vi "Wait Single With Memory.vi"(8 "error in (no error)":errorcluster, 9 "Timeout in ms (-1)":i32=-1, 10 "Ignore previous (F)":bool, 11 "Notifier in":refnum<class "Notifier.lvclass">) -> (0 "error out":errorcluster, 1 "Timed out?":bool, 2 "Data Notification":refnum<class "Data.lvclass">, 3 "Notifier out":refnum<class "Notifier.lvclass">)   [LabVIEW 2020, in "Data.lvlib" / "Notifier.lvclass"]
doc: "Wait on notification from a single notifier with notifier history."
uses:
  Notifier.lvclass
  Data.lvclass
  Notifier.lvclass/Notifier.ctl
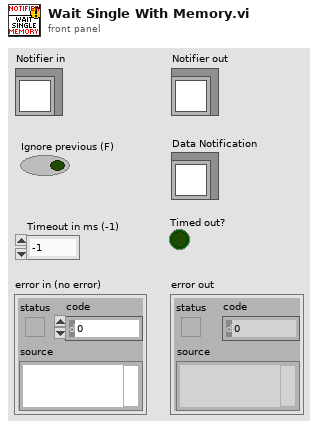
[diagram p1: front panel]
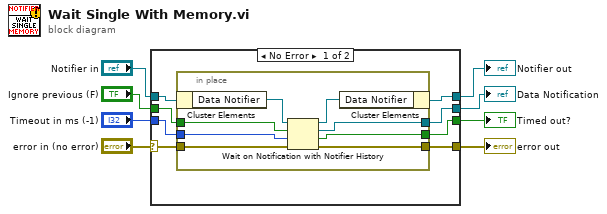
[diagram p0: block diagram]
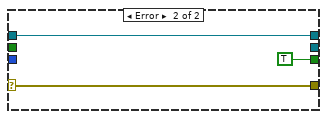
[diagram p2: hidden frame]
diagram:
  n1 = case shown="No Error" "error in (no error)" {
    selector: "error in (no error)" -> [w14 w27]
    tunnel: [w13 w27] -> w7
    tunnel: [w15 w26] -> w5
    tunnel: "Notifier in" -> [w16 w26]
    tunnel: [w12 _] -> w4
    tunnel: "Timeout in ms (-1)" -> [w11 _]
    tunnel: "Ignore previous (F)" -> [w10 _]
    tunnel: [w9 TRUE ("timed out?")] -> w1
    frame No Error {
      n2 = in-place {
        in-place-border: w14 -> [w20]
        in-place-border: [w22] -> w13
        in-place-border: [w21] -> w12
        in-place-border: w11 -> [w19]
        in-place-border: w10 -> [w18]
        in-place-border: [w17] -> w9
        n3 = in-place-cluster #1(w16) -> ("Data Notifier"=w24:refnum<notifier>)
        n4 = Wait on Notification with Notifier History(0:w24, 1:w18, 2:w19, 3:w20) -> (8:w23:refnum<notifier>, 9:w21:refnum<class "Data.lvclass">, 10:w17:bool, 11:w22:errorcluster)
        n5 = in-place-cluster #1("Data Notifier"=w23) -> (w15:refnum<class "Notifier.lvclass">)
      }
    }
    frame Error {
    }
  }
  "error out" <- w7
  "Notifier out" <- w5
  "Data Notification" <- w4
  "Timed out?" <- w1
